vi "utility.DelayTime.Short.vi"(11 "Timer":u32=3) -> ()   [LabVIEW 2012, in "Lib_UEL.ATE.lvlib" / "Lib_App.lvlib"]
uses:
  Lib_App.lvlib
panel:
  out "错误输出":errorcluster
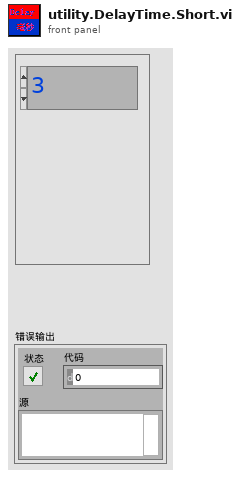
[diagram p1: front panel]
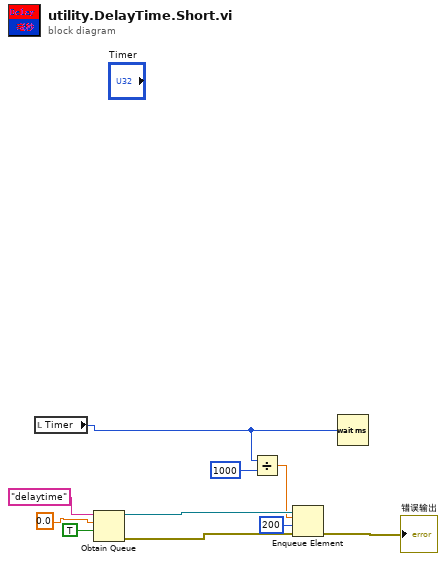
[diagram p0: block diagram]
diagram:
  n1 = local read "Timer"() -> (w5:u32)
  n2 = Obtain Queue(name (unnamed)="delaytime" ("名称（未命名）"), element data type=0.0 ("y"), create if not found? (T)=TRUE ("如未找到是否创建？(T)")) -> (queue out=w7:refnum<queue>, error out=w6:errorcluster)  [unwired: 2 in, 1 out]
  n3 = Divide(x=w5, y=u32 1000) -> (x/y=w1:dbl)
  n4 = Enqueue Element(queue=w7, element=w1, timeout in ms (-1)=200 ("超时毫秒(-1)"), error in (no error)=w6) -> (error out=→"错误输出":errorcluster)  [unwired: 2 out]
  n5 = Wait (ms)(milliseconds to wait=w5) -> ()  [unwired: 1 out]
